vi "Clear Faults.vi"(1 "Initialize":bool=TRUE, 5 "ES System Data":T4={"Voltage"=0.0, "Current"=0.0, "SOC Avg"=0.0, "Faults"=0, "Alarms"=0, "# Strings"=0, "Max Temp"=0, "Min Temp"=0, "Max Cell Voltage"=0.0, "Min Cell Voltage"=0.0, "Energy Capacity"=0.0, "Energy Remaining"=0.0, "SOC Min"=0.0, "SOC Max"=0.0, "ES Fault"=FALSE, "String Select"=enum."3 Strings", "ES Com Fault"=FALSE, "SOH Avg"=0.0}, 7 "PC Data":T2 {"Alarms 2" format="%016b"; "Faults 2" format="%016b"; "Alarms 1" format="%016b"; "Faults 1" format="%016b"; "Contactor FB" format="%.0b"; "DC Voltage SP" format="%2.1f"; "Clear Faults SP" format="%.0b"; "Neutral Current" format="%2.1f"; "AC Current - L2" format="%2.1f"; "AC Voltage - L2" format="%2.1f"; "Temperature" format="%2.1f"; "DC Voltage" format="%2.1f"; "AC Current SP" format="%2.1f"; "AC Voltage SP" format="%2.1f"; "Frequency SP" format="%2.1f"; "AC Frequency" format="%2.1f"; "AC Current - L1" format="%2.1f"; "AC Voltage- L1" format="%2.1f"}, 9 "FPGA Data":T1 {"SSG Active Current" format="%2.1f"; "PV Reactive Power (L1)" format="%2.1f"; "PV Reactive Power (L2)" format="%2.1f"; "PV Total Reactive Power" format="%2.1f"; "Gen Reactive Power (L1)" format="%2.1f"; "Gen Reactive Power (L2)" format="%2.1f"; "Gen Total Reactive Power" format="%2.1f"; "SSG Reactive Power (L1)" format="%2.1f"; "SSG Reactive Power (L2)" format="%2.1f"; "SSG Total Reactive Power" format="%2.1f"; "PV Total Current" format="%2.1f"; "PV Total Voltage" format="%2.1f"; "PV Active Power (L1)" format="%2.1f"; "PV Active Power (L2)" format="%2.1f"; "PV App Power (L1)" format="%2.1f"; "PV App Power (L2)" format="%2.1f"; "PV Total Active Power" format="%2.1f"; "PV Total App Power" format="%2.1f"; "PV Arms (L1)" format="%2.1f"; "PV Arms (L2)" format="%2.1f"; "PV Vrms (L1)" format="%2.1f"; "PV Vrms (L2)" format="%2.1f"; "Gen Total Current" format="%2.1f"; "SSG Total Current" format="%2.1f"; "Gen Total Voltage" format="%2.1f"; "SSG Total Voltage" format="%2.1f"; "Gen Active Power (L1)" format="%2.1f"; "Gen Active Power (L2)" format="%2.1f"; "SSG Active Power (L1)" format="%2.1f"; "SSG Active Power (L2)" format="%2.1f"; "Gen App Power (L1)" format="%2.1f"; "Gen App Power (L2)" format="%2.1f"; "SSG App Power (L1)" format="%2.1f"; "SSG App Power (L2)" format="%2.1f"; "Gen Total Active Power" format="%2.1f"; "Gen Total App Power" format="%2.1f"; "Gen Arms (L1)" format="%2.1f"; "Gen Arms (L2)" format="%2.1f"; "Gen Vrms (L1)" format="%2.1f"; "Gen Vrms (L2)" format="%2.1f"; "SSG Total Active Power" format="%2.1f"; "SSG Total App Power" format="%2.1f"; "SSG Arms (L1)" format="%2.1f"; "SSG Arms (L2)" format="%2.1f"; "SSG Vrms (L1)" format="%2.1f"; "SSG Vrms (L2)" format="%2.1f"}, 11 "Error In":errorcluster) -> (3 "Wait for Fault":bool, 8 "Clear Error":bool, 15 "Error Out":errorcluster)   [LabVIEW 2014]
doc: "This code will pulse the fault clear signal for 3 seconds once every 15 minutes. If any fault persists for 30 seconds after the fault clear signal is sent, a counter will increment. If the counter reaches 3, the Manual Shutdown bit will be set high. Controller reboot necessary to reset."
uses:
  Controls/ES System Data.ctl
  Controls/StringSelector.ctl
  Controls/PC Data.ctl
  Controls/MicroZed Config Op Mode.ctl
  Controls/FPGA Data.ctl
panel:
  in  "PC CMD":bool=TRUE
  out "Attempt Counter":i16
  in  "Pulse On Time":u32=3
  in  "Pulse Off Time":u32=20
  in  "Wait for Fault Time":dbl=10.0 caption="Time Target (s)"
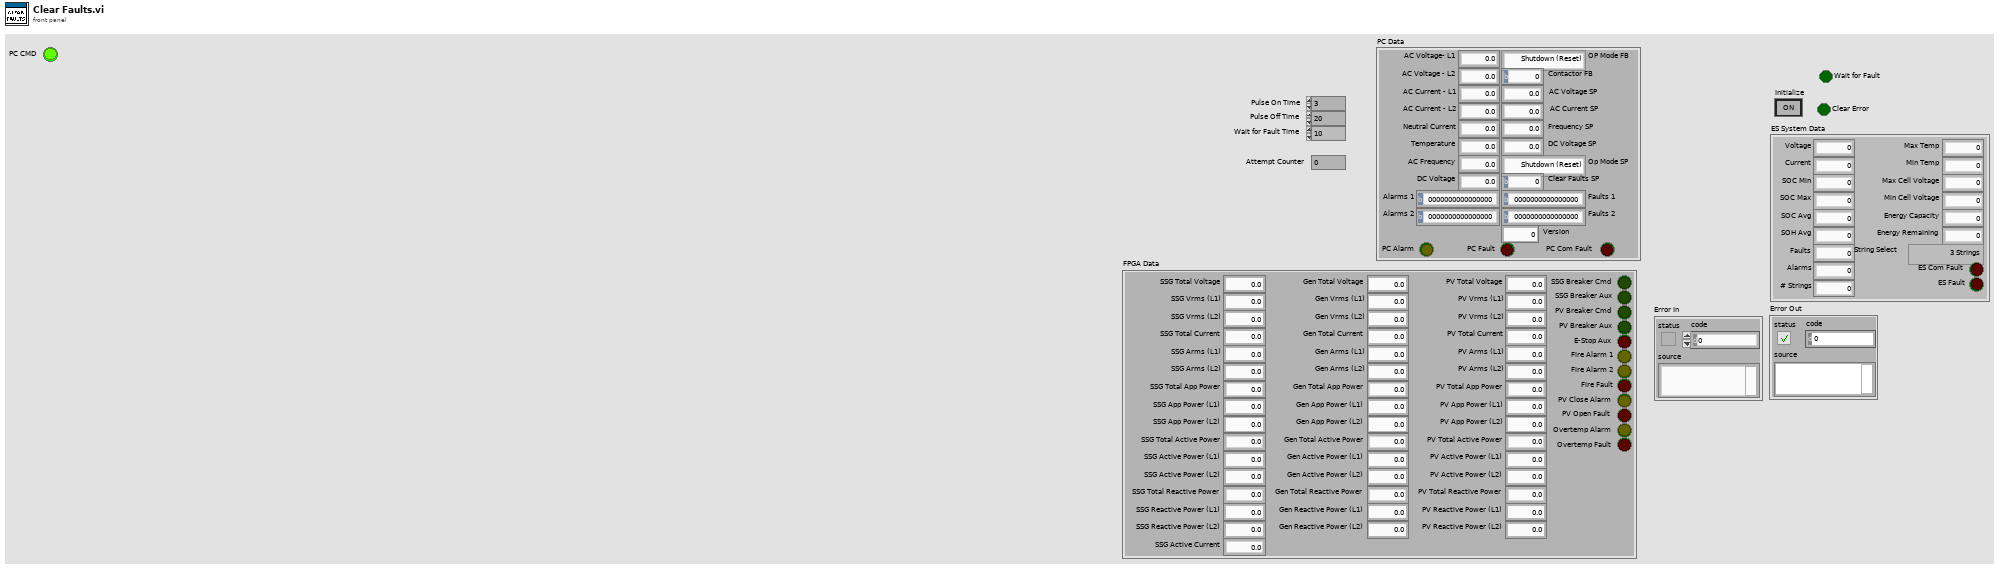
[diagram p1: front panel]
types:
  T1 = typedef "FPGA Data.ctl" = cluster{"Gen Total Voltage":dbl, "Gen Vrms (L1)":dbl, "Gen Vrms (L2)":dbl, "Gen Total Current":dbl, "Gen Arms (L1)":dbl, "Gen Arms (L2)":dbl, "Gen Total App Power":dbl, "Gen App Power (L1)":dbl, "Gen App Power (L2)":dbl, "Gen Total Active Power":dbl, "Gen Active Power (L1)":dbl, "Gen Active Power (L2)":dbl, "Gen Total Reactive Power":dbl, "Gen Reactive Power (L1)":dbl, "Gen Reactive Power (L2)":dbl, "SSG Total Voltage":dbl, "SSG Vrms (L1)":dbl, "SSG Vrms (L2)":dbl, "SSG Total Current":dbl, "SSG Arms (L1)":dbl, "SSG Arms (L2)":dbl, "SSG Total App Power":dbl, "SSG App Power (L1)":dbl, "SSG App Power (L2)":dbl, "SSG Total Active Power":dbl, "SSG Active Power (L1)":dbl, "SSG Active Power (L2)":dbl, "SSG Total Reactive Power":dbl, "SSG Reactive Power (L1)":dbl, "SSG Reactive Power (L2)":dbl, "PV Total Voltage":dbl, "PV Vrms (L1)":dbl, "PV Vrms (L2)":dbl, "PV Total Current":dbl, "PV Arms (L1)":dbl, "PV Arms (L2)":dbl, "PV Total App Power":dbl, "PV App Power (L1)":dbl, "PV App Power (L2)":dbl, "PV Total Active Power":dbl, "PV Active Power (L1)":dbl, "PV Active Power (L2)":dbl, "PV Total Reactive Power":dbl, "PV Reactive Power (L1)":dbl, "PV Reactive Power (L2)":dbl, "SSG Breaker Cmd":bool, "SSG Breaker Aux":bool, "PV Breaker Cmd":bool, "PV Breaker Aux":bool, "E-Stop Aux":bool, "Fire Alarm 1":bool, "Fire Alarm 2":bool, "Fire Fault":bool, "PV Close Alarm":bool, "SSG Active Current":dbl, "Overtemp Alarm":bool, "Overtemp Fault":bool, "PV Open Fault":bool}
  T2 = typedef "PC Data.ctl" = cluster{"AC Voltage- L1":dbl, "AC Voltage - L2":dbl, "AC Current - L1":dbl, "AC Current - L2":dbl, "Neutral Current":dbl, "Temperature":dbl, "AC Frequency":dbl, "DC Voltage":dbl, "AC Voltage SP":dbl, "AC Current SP":dbl, "Frequency SP":dbl, "Op Mode SP":T3, "Clear Faults SP":u16, "PC Com Fault":bool, "PC Fault":bool, "DC Voltage SP":dbl, "OP Mode FB":T3, "Contactor FB":u16, "Faults 1":u16, "Alarms 1":u16, "Faults 2":u16, "Alarms 2":u16, "PC Alarm":bool, "Version":u16}
  T3 = typedef "MicroZed Config Op Mode.ctl" = enum16{"Shutdown (Reset)", "Startup", "Idle", "Voltage Mode", "Current Mode", "Fault", "OL Voltage (Debug)", "No Data"}
  T4 = typedef "ES System Data.ctl" = cluster{"Voltage":sgl, "Current":sgl, "SOC Avg":sgl, "Faults":u16, "Alarms":u16, "# Strings":u16, "Max Temp":i16, "Min Temp":i16, "Max Cell Voltage":sgl, "Min Cell Voltage":sgl, "Energy Capacity":sgl, "Energy Remaining":sgl, "SOC Min":sgl, "SOC Max":sgl, "ES Fault":bool, "String Select":T5, "ES Com Fault":bool, "SOH Avg":sgl}
  T5 = typedef "StringSelector.ctl" = enum16{"1 String (1)", "1 String (2)", "1 String (3)", "2 Strings (1 2)", "2 Strings (2 3)", "2 Strings (1 3)", "3 Strings"}
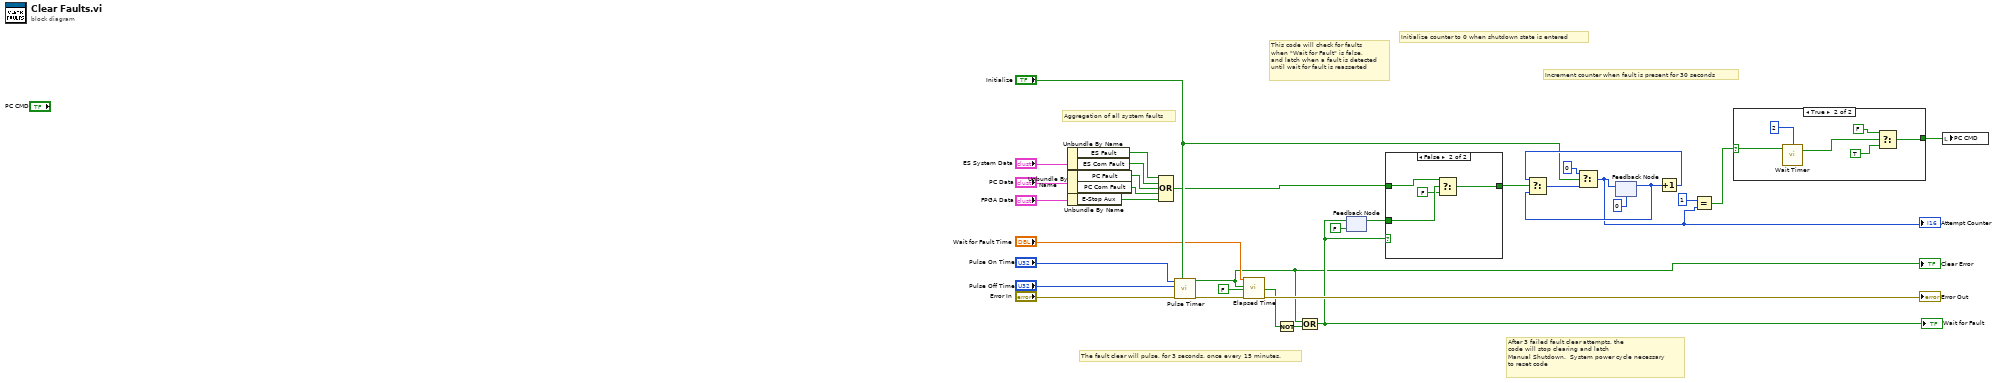
[diagram p0: block diagram]
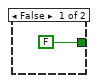
[diagram p2: hidden frame]
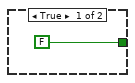
[diagram p3: hidden frame]
diagram:
  # "Increment counter when fault is present for 30 seconds"
  # "Initialize counter to 0 when shutdown state is entered"
  # "The fault clear will pulse, for 3 seconds, once every 15 minutes."
  # "After 3 failed fault clear attempts, the \ncode will stop clearing and latch \nManual Shutdown.  System power cycle necessary\nto reset code"
  # "This code will check for faults\nwhen \"Wait for Fault\" is false,\nand latch when a fault is detected\nuntil wait for fault is reasserted"
  # "Aggregation of all system faults"
  n1 = Unbundle By Name("ES System Data") -> ("ES Fault"=w24:bool, "ES Com Fault"=w25:bool)
  n2 = Unbundle By Name("PC Data") -> ("PC Fault"=w26:bool, "PC Com Fault"=w27:bool)
  n3 = Unbundle By Name("FPGA Data") -> ("E-Stop Aux"=w28:bool)
  n4 = Compound Arithmetic op=OR(w24, w25, w26, w27, w28) -> (w10:bool)
  n5 = call "Pulse Timer.vi"("Initialize"="Initialize", "Error In"="Error In", "Off Time"="Pulse Off Time", "On Time"="Pulse On Time") -> ("Error Out"=w18:errorcluster, "Boolean Out"=w1:bool)  [unwired: 6 in]
  "Clear Error" <- w1
  n6 = call "Elapsed Time"("Time Target (s)"="Wait for Fault Time", "Reset"=w1, "Auto Reset"=FALSE, "error in (no error)"=w18) -> ("Time has Elapsed"=w16:bool, "error out"=→"Error Out":errorcluster)  [unwired: 8 in, 6 out]
  n7 = Not(x=w16) -> (.not. x?=w15:bool)
  n8 = Compound Arithmetic op=OR(w1, w15) -> (w8:bool)
  "Wait for Fault" <- w8
  n9 = feedback #1(FALSE) -> (w6:bool)
  n10 = feedback-in #1(w8) -> ()
  n11 = case shown="False" w8 {
    tunnel: w10 -> [_ w35]
    tunnel: [FALSE w37] -> w9
    tunnel: w6 -> [_ w38]
    frame True {
    }
    frame False {
      n12 = Select(t=w35, s=w38, f=FALSE ("t")) -> (s? t:f=w37:bool)
    }
  }
  n13 = feedback #2(i16 0) -> (w20:i16)
  n14 = Increment(x=w20) -> (x+1=w21:i16)
  n15 = Select(t=w21, s=w9, f=w20) -> (s? t:f=w11:i16)
  n16 = Select(t=i16 0, s="Initialize", f=w11) -> (s? t:f=w4:i16)
  "Attempt Counter" <- w4
  n17 = feedback-in #2(w4) -> ()
  n18 = Equal?(x=u16 1, y=w4) -> (x = y?=w3:bool)
  n19 = case shown="True" w3 {
    selector: w3 -> [_ w44]
    tunnel: [FALSE w40] -> w2
    frame False {
    }
    frame True {
      n20 = call "Wait Timer.vi"("Boolean In"=w44, "Timer"=u32 2) -> ("Boolean Out"=w43:bool)  [unwired: 3 in]
      n21 = Select(t=FALSE, s=w43, f=TRUE) -> (s? t:f=w40:bool)
    }
  }
  n22 = local write "PC CMD"(w2) -> ()
